vi "4Pi DCM - Crop Image.vi"(9 "ROI Size":i32=3, 10 "Image Refs":T1[](array[typedef]), 11 "Input Image (U16)":u16[][](array[numeric])) -> (3 "Output Image Stack":u16[][][](array[numeric]))   [LabVIEW 2016]
uses:
  <vilib>/vision/Image Controls.llb/IMAQ Image.ctl
  Display Module/Display Module Custom Controls/ROI Descriptor.ctl
panel:
  out "Numeric":i32
  out "ROI4":u16[][](graph)
  out "ROI3":u16[][](graph)
  out "ROI2":u16[][](graph)
  out "ROI1":u16[][](graph)
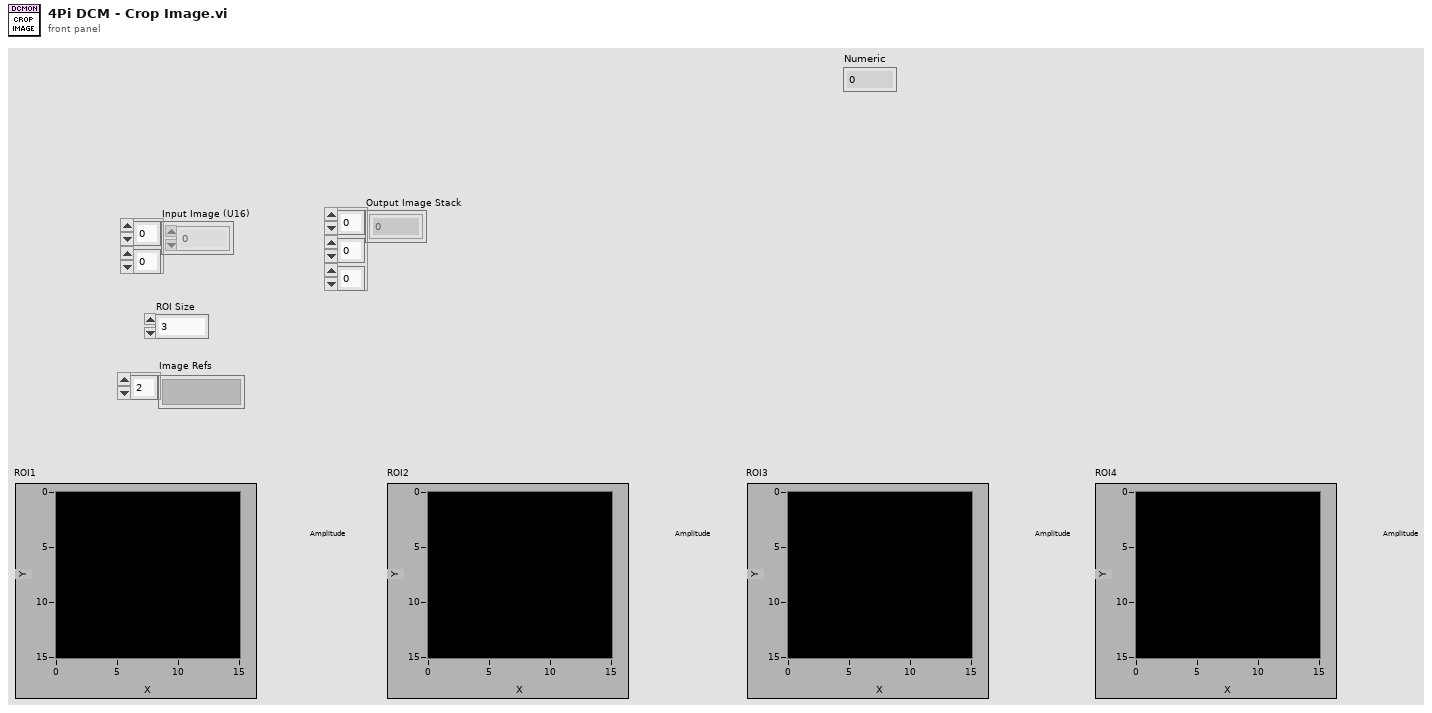
[diagram p1: front panel]
types:
  T1 = typedef "IMAQ Image.ctl" = refnum<image>
  T2 = typedef "ROI Descriptor.ctl" = cluster{"Global Rectangle":i32[], "Contours":cluster{"Contour Type":u32, "ROI Type":u32, "Points":i32[]}[]}
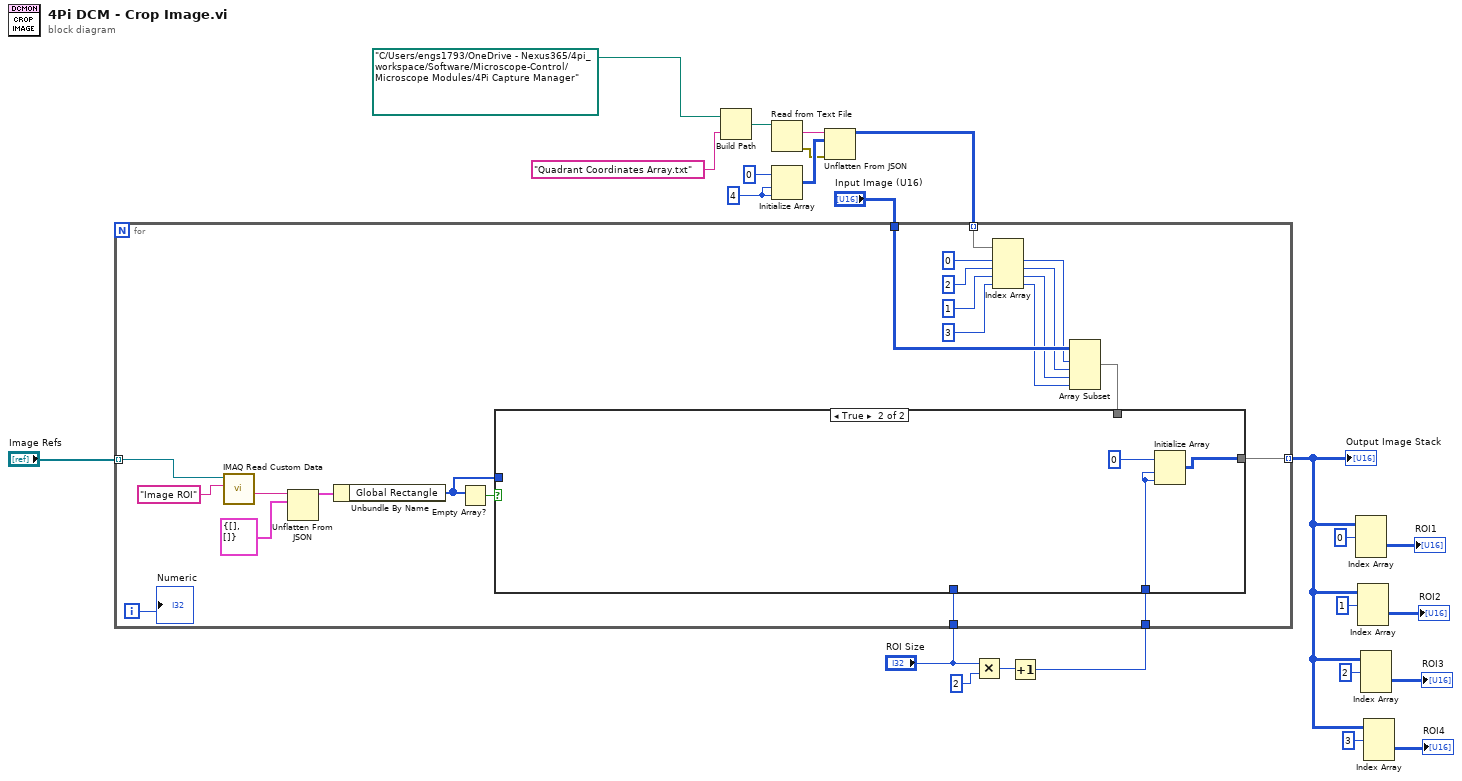
[diagram p0: block diagram]
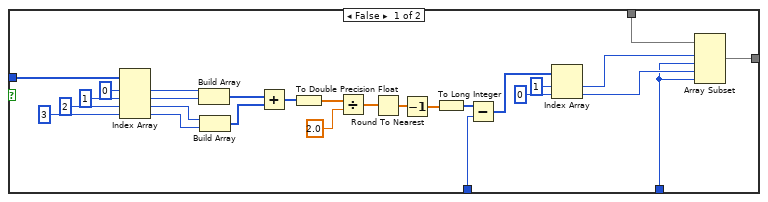
[diagram p2: hidden frame]
diagram:
  w18 = 4 ("dimension size")
  n1 = Build Path(base path=path "C:/Users/engs1793/OneDrive - Nexus365/4pi_workspace/Software/Microscope-Control/Microscope Modules/4Pi Capture Manager" ("path"), name or relative path="Quadrant Coordinates Array.txt") -> (appended path=w21:path)
  n2 = Read from Text File(file (use dialog)=w21) -> (text=w20:string, error out=w19:errorcluster)  [unwired: 3 in, 2 out]
  n3 = Initialize Array(0 ("element"), w18, w18) -> (w22:i32[][])
  n4 = Unflatten From JSON(JSON string=w20, type and defaults=w22, error in (no error)=w19) -> (value=w1:i32[][])  [unwired: 4 in, 1 out]
  n5 = Multiply(x="ROI Size", y=2) -> (x*y=w15:i32)
  n6 = Increment(x=w15) -> (x+1=w14:i32)
  n7 = for {
    tunnel: "Input Image (U16)" -> [w46]
    tunnel: w14 -> [w30]
    tunnel: "ROI Size" -> [w29]
    tunnel: [w28] -> w3 mode=indexing
    tunnel: "Image Refs" -> [w27] mode=indexing
    tunnel: w1 -> [w25] mode=indexing
    i -> [w26]
    n8 = call "IMAQ Read Custom Data"("Key"="Image ROI", "Image"=w27) -> ("Custom Data Out"=w35:string)  [unwired: 7 in, 2 out]
    n9 = Unflatten From JSON(JSON string=w35, type and defaults=T2 {"Global Rectangle"=[], "Contours"=[]} ("Image ROI Descriptor")) -> (value=w33:T2)  [unwired: 5 in, 1 out]
    n10 = Unbundle By Name(w33) -> ("Global Rectangle"=w31:i32[])
    n11 = Empty Array?(array=w31) -> (empty?=w32:bool)
    n12 = Index Array(array=w25, index #1=0 ("index"), index #2=2 ("index"), index #3=1 ("index"), index #4=3 ("index")) -> (element #1=w44:i32, element #2=w43:i32, element #3=w39:i32, element #4=w38:i32)
    n13 = Array Subset(array=w46, index (row)=w44, length (row)=w43, index (col)=w39, length (col)=w38) -> (w37:u16[][])
    n14 = case shown="True" w32 {
      tunnel: w37 -> [w53 _]
      tunnel: [w52 w74] -> w28
      tunnel: w31 -> [w51 _]
      tunnel: w30 -> [w50 w75]
      tunnel: w29 -> [w49 _]
      frame False {
        n15 = Index Array(array=w51, index #1=0 ("index"), index #2=1 ("index"), index #3=2 ("index"), index #4=3 ("index")) -> (element #1=w66:i32, element #2=w65:i32, element #3=w64:i32, element #4=w63:i32)
        n16 = Build Array(w66, w65) -> (w62:i32[])
        n17 = Build Array(w64, w63) -> (w61:i32[])
        n18 = Add(x=w62, y=w61) -> (x+y=w68:i32[])
        n19 = To Double Precision Float(number=w68) -> (double precision float=w69:dbl[])
        n20 = Divide(x=w69, y=2.0) -> (x/y=w60:dbl[])
        n21 = Round To Nearest(number=w60) -> (nearest integer value=w48:dbl[])
        n22 = Decrement(x=w48) -> (x-1=w47:dbl[])
        n23 = To Long Integer(number=w47) -> (32bit integer=w59:i32[])
        n24 = Subtract(x=w59, y=w49) -> (x-y=w58:i32[])
        n25 = Index Array(array=w58, index #1=1 ("index"), index #2=0 ("index")) -> (element #1=w55:i32, element #2=w54:i32)
        n26 = Array Subset(array=w53, index (row)=w55, length (row)=w50, index (col)=w54, length (col)=w50) -> (w52:u16[][])
      }
      frame True {
        n27 = Initialize Array(u16 0, w75, w75) -> (w74:u16[][])
      }
    }
    "Numeric" <- w26
  }
  "Output Image Stack" <- w3
  n28 = Index Array(array=w3, index (dim 0)=0 ("index (page)")) -> (element=→"ROI1":u16[][])  [unwired: 2 in]
  n29 = Index Array(array=w3, index (dim 0)=1 ("index (page)")) -> (element=→"ROI2":u16[][])  [unwired: 2 in]
  n30 = Index Array(array=w3, index (dim 0)=2 ("index (page)")) -> (element=→"ROI3":u16[][])  [unwired: 2 in]
  n31 = Index Array(array=w3, index (dim 0)=3 ("index (page)")) -> (element=→"ROI4":u16[][])  [unwired: 2 in]
